vi "InitializeOpStates.vi"(9 "metric ids":string[](array[string]), 10 "op state in":T5) -> (1 "valid config":bool, 2 "conv op state":T1)   [LabVIEW 2017, in "Trigger.lvlib"]
uses:
  <vilib>/addons/InsightCM/Devices/Shared/Common/Trigger/Trigger.lvlib
  <vilib>/addons/InsightCM/MessageBus/Base/controls/OperatingState.ctl
  <vilib>/addons/InsightCM/MessageBus/Base/controls/KeyValuePair.ctl
  <vilib>/addons/InsightCM/MessageBus/Base/controls/Trigger.ctl
  <vilib>/addons/InsightCM/MessageBus/Base/controls/Condition.ctl
  <vilib>/addons/InsightCM/Devices/Shared/Common/Trigger/controls/TriggerOperatingState.ctl
  <vilib>/addons/InsightCM/Devices/Shared/Common/Trigger/controls/TriggerCondition.ctl
  <vilib>/addons/InsightCM/Utilities/DeviceModelHelpers/DeviceModelHelpers.lvlib
  <vilib>/addons/InsightCM/Devices/Shared/Common/OpState/OpState.lvlib
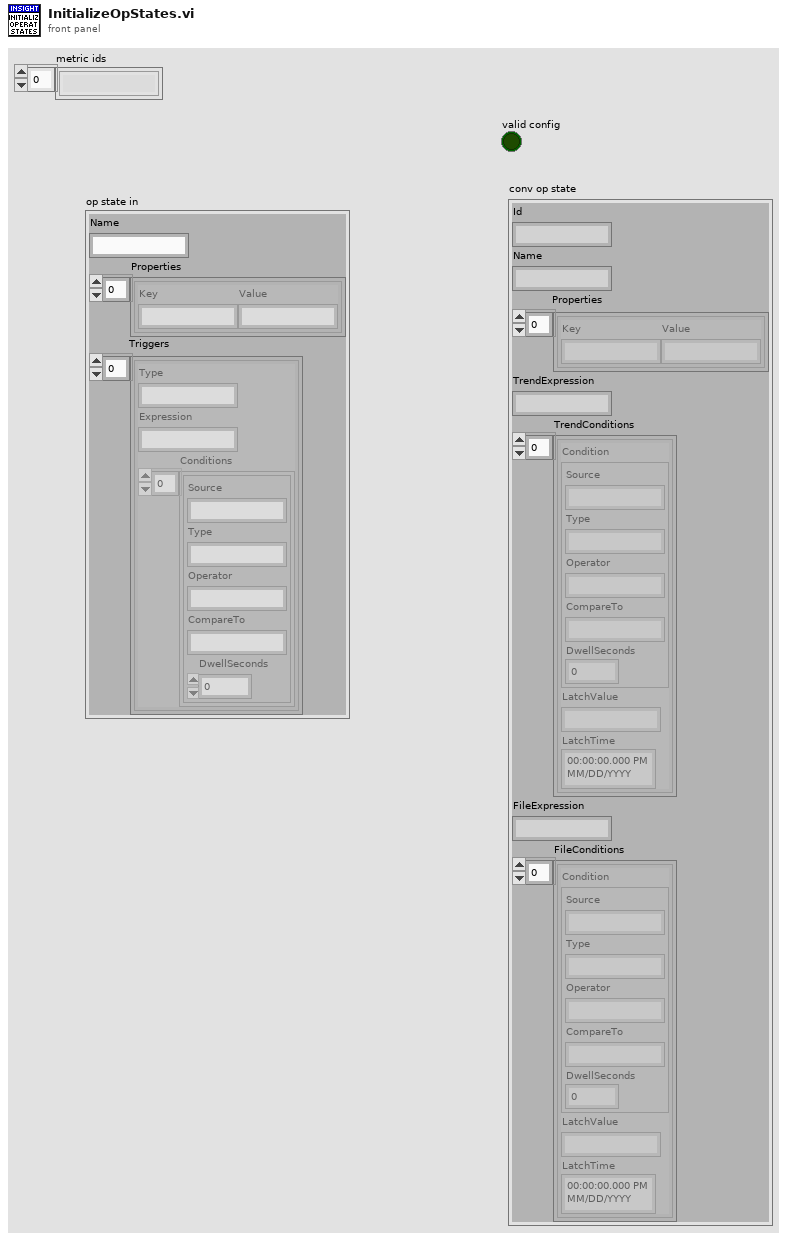
[diagram p1: front panel]
types:
  T1 = typedef "Trigger.lvlib/TriggerOperatingState.ctl" = cluster{"Id":string, "Name":string, "Properties":T2[], "TrendExpression":string, "TrendConditions":T3[], "FileExpression":string, "FileConditions":T3[]}
  T2 = typedef "KeyValuePair.ctl" = cluster{"Key":string, "Value":string}
  T3 = typedef "Trigger.lvlib/TriggerCondition.ctl" = cluster{"Condition":T4, "LatchValue":string, "LatchTime":timestamp}
  T4 = typedef "Condition.ctl" = cluster{"Source":string, "Type":string, "Operator":string, "CompareTo":string, "DwellSeconds":dbl}
  T5 = typedef "OperatingState.ctl" = cluster{"Name":string, "Properties":T2[], "Triggers":T6[]}
  T6 = typedef "Trigger.ctl" = cluster{"Type":string, "Expression":string, "Conditions":T4[]}
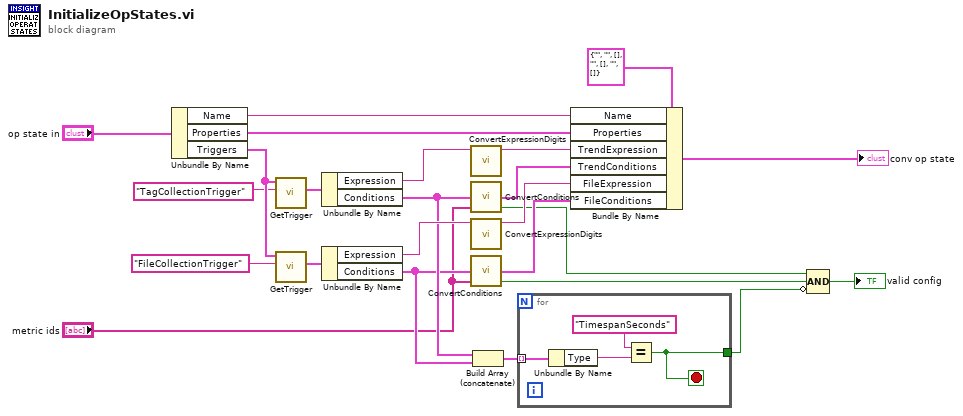
[diagram p0: block diagram]
diagram:
  n1 = Unbundle By Name("op state in") -> ("Name"=w23:string, "Properties"=w22:T2[], "Triggers"=w17:T6[])
  n2 = call <vilib>:"GetTrigger.vi"("type"="TagCollectionTrigger", "triggers"=w17) -> ("trigger"=w19:T6)  [unwired: 8 in, 1 out]
  n3 = call <vilib>:"GetTrigger.vi"("type"="FileCollectionTrigger", "triggers"=w17) -> ("trigger"=w18:T6)  [unwired: 8 in, 1 out]
  n4 = Unbundle By Name(w19) -> ("Expression"=w12:string, "Conditions"=w8:T4[])
  n5 = Unbundle By Name(w18) -> ("Expression"=w10:string, "Conditions"=w7:T4[])
  n6 = call <vilib>:"ConvertExpressionDigits.vi"("input"=w12) -> ("output"=w11:string)  [unwired: 10 in]
  n7 = call <vilib>:"ConvertConditions.vi"("metric ids"="metric ids", "conditions"=w8) -> ("valid config"=w2:bool, "trigger conditions"=w21:T3[])  [unwired: 2 in]
  n8 = call <vilib>:"ConvertExpressionDigits.vi"("input"=w10) -> ("output"=w9:string)  [unwired: 10 in]
  n9 = call <vilib>:"ConvertConditions.vi"("metric ids"="metric ids", "conditions"=w7) -> ("valid config"=w1:bool, "trigger conditions"=w20:T3[])  [unwired: 2 in]
  n10 = Build Array (concatenate)(w8, w7) -> (w6:T4[])
  n11 = for {
    tunnel: w6 -> [w28] mode=indexing
    tunnel: [w25] -> w5
    stop <- w25 stop-if-true
    n12 = Unbundle By Name(w28) -> ("Type"=w27:string)
    n13 = Equal?(x="TimespanSeconds", y=w27) -> (x = y?=w25:bool)
  }
  n14 = Bundle By Name(cluster=T1 {"Id"="", "Name"="", "Properties"=[], "TrendExpression"="", "TrendConditions"=[], "FileExpression"="", "FileConditions"=[]} ("OperatingState"), "Name"=w23, "Properties"=w22, "TrendExpression"=w11, "TrendConditions"=w21, "FileExpression"=w9, "FileConditions"=w20) -> (→"conv op state":T1)
  n15 = Compound Arithmetic op=AND(w2, w1, invert w5) -> (→"valid config":bool)
